vi "Get_Data_With_Condition.vi"(8 "error in (no error)":errorcluster caption="entrée d'erreur (pas d'erreur)", 11 "Firebase Benches en entrée":refnum<class "Firebase Benches P2193.lvclass">) -> (0 "error out":errorcluster caption="sortie d'erreur", 3 "Firebase Benches en sortie":refnum<class "Firebase Benches P2193.lvclass">)   [LabVIEW 2020, in "Library Instrument & Equipement.lvlib" / "Library FireBase.lvlib" / "Firebase Benches P2193.lvclass"]
doc: "Returns data according to Value_To_Find on Collection_to_find Use Nb_To_Read to determine the number to read\nPlease initialise the following values before use the VI\n - Name BDD\n - Value to find\n - API Key\n - Field Filter\n - Field Order\n - Collection_to_find\n\nIf there is no Field order -> Field Order=Field Filter"
uses:
  Firebase Benches P2193.lvclass
  C:/Users/ngarcin/OneDrive - Altyor/Standard TB/Class/Firebase/Source/Firebase Altyor/Firebase Altyor.lvclass
  C:/Users/ngarcin/OneDrive - Altyor/Standard TB/Class/Firebase/Source/Firebase Driver/Firebase Driver.lvclass
  Firebase Benches P2193.lvclass/Firebase Benches P2193.ctl
  JSON API/JSON Value/Set from JSON string.vi
  JSON API/JSON Value/JSON Value.lvclass
  Firebase Altyor/Firebase Altyor.lvclass
  JSON API/Variant JSON/Variant JSON.lvlib
  JSON API/Get Polymorphic/JSON GetSet.lvlib
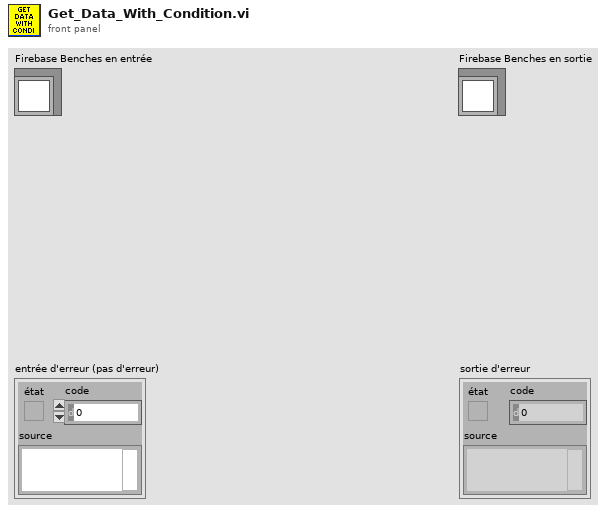
[diagram p1: front panel]
types:
  T1 = cluster{"name":string, "fields":cluster{"Result":cluster{"booleanValue":bool}, "CreationDate":cluster{"timestampValue":string}, "Batch":cluster{"stringValue":string}, "SerialNumber":cluster{"stringValue":string}, "EndOfProduction":cluster{"timestampValue":string}, "FW_Version":cluster{"mapValue":cluster{"fields":cluster{"Bootloader":cluster{"mapValue":cluster{"fields":cluster{"File_Name":cluster{"stringValue":string}, "Version":cluster{"mapValue":cluster{"fields":cluster{"Major":cluster{"stringValue":string}, "Minor":cluster{"stringValue":string}}}}, "Checksum":cluster{"stringValue":string}}}}, "SoftDevice":cluster{"mapValue":cluster{"fields":cluster{"File_Name":cluster{"stringValue":string}, "Version":cluster{"mapValue":cluster{"fields":cluster{"Major":cluster{"stringValue":string}, "Minor":cluster{"stringValue":string}}}}, "Checksum":cluster{"stringValue":string}}}}, "DFU":cluster{"mapValue":cluster{"fields":cluster{"File_Name":cluster{"stringValue":string}, "Version":cluster{"mapValue":cluster{"fields":cluster{"Major":cluster{"stringValue":string}, "Minor":cluster{"stringValue":string}}}}, "Checksum":cluster{"stringValue":string}}}}}}}, "PartNumber":cluster{"stringValue":string}, "OrderNumber":cluster{"stringValue":string}, "Operator":cluster{"stringValue":string}, "SN_CPU":cluster{"stringValue":string}}}[]
  T2 = cluster{"name":string, "fields":cluster{"Result":cluster{"booleanValue":bool}, "CreationDate":cluster{"timestampValue":string}, "Batch":cluster{"stringValue":string}, "SerialNumber":cluster{"stringValue":string}, "EndOfProduction":cluster{"timestampValue":string}, "FW_Version":cluster{"mapValue":cluster{"fields":cluster{"Bootloader":cluster{"mapValue":cluster{"fields":cluster{"File_Name":cluster{"stringValue":string}, "Version":cluster{"mapValue":cluster{"fields":cluster{"Major":cluster{"stringValue":string}, "Minor":cluster{"stringValue":string}}}}, "Checksum":cluster{"stringValue":string}}}}, "SoftDevice":cluster{"mapValue":cluster{"fields":cluster{"File_Name":cluster{"stringValue":string}, "Version":cluster{"mapValue":cluster{"fields":cluster{"Major":cluster{"stringValue":string}, "Minor":cluster{"stringValue":string}}}}, "Checksum":cluster{"stringValue":string}}}}, "DFU":cluster{"mapValue":cluster{"fields":cluster{"File_Name":cluster{"stringValue":string}, "Version":cluster{"mapValue":cluster{"fields":cluster{"Major":cluster{"stringValue":string}, "Minor":cluster{"stringValue":string}}}}, "Checksum":cluster{"stringValue":string}}}}}}}, "PartNumber":cluster{"stringValue":string}, "OrderNumber":cluster{"stringValue":string}, "Operator":cluster{"stringValue":string}, "SN_CPU":cluster{"stringValue":string}}}
  T3 = cluster{"document":cluster{"name":string, "fields":cluster{"Result":cluster{"booleanValue":bool}, "CreationDate":cluster{"timestampValue":string}, "Batch":cluster{"stringValue":string}, "SerialNumber":cluster{"stringValue":string}, "EndOfProduction":cluster{"timestampValue":string}, "FW_Version":cluster{"mapValue":cluster{"fields":cluster{"Bootloader":cluster{"mapValue":cluster{"fields":cluster{"File_Name":cluster{"stringValue":string}, "Version":cluster{"mapValue":cluster{"fields":cluster{"Major":cluster{"stringValue":string}, "Minor":cluster{"stringValue":string}}}}, "Checksum":cluster{"stringValue":string}}}}, "SoftDevice":cluster{"mapValue":cluster{"fields":cluster{"File_Name":cluster{"stringValue":string}, "Version":cluster{"mapValue":cluster{"fields":cluster{"Major":cluster{"stringValue":string}, "Minor":cluster{"stringValue":string}}}}, "Checksum":cluster{"stringValue":string}}}}, "DFU":cluster{"mapValue":cluster{"fields":cluster{"File_Name":cluster{"stringValue":string}, "Version":cluster{"mapValue":cluster{"fields":cluster{"Major":cluster{"stringValue":string}, "Minor":cluster{"stringValue":string}}}}, "Checksum":cluster{"stringValue":string}}}}}}}, "PartNumber":cluster{"stringValue":string}, "OrderNumber":cluster{"stringValue":string}, "Operator":cluster{"stringValue":string}, "SN_CPU":cluster{"stringValue":string}}}}
  T4 = cluster{"document":cluster{"name":string, "fields":cluster{"Result":cluster{"booleanValue":bool}, "CreationDate":cluster{"timestampValue":string}, "Batch":cluster{"stringValue":string}, "SerialNumber":cluster{"stringValue":string}, "EndOfProduction":cluster{"timestampValue":string}, "FW_Version":cluster{"mapValue":cluster{"fields":cluster{"Bootloader":cluster{"mapValue":cluster{"fields":cluster{"File_Name":cluster{"stringValue":string}, "Version":cluster{"mapValue":cluster{"fields":cluster{"Major":cluster{"stringValue":string}, "Minor":cluster{"stringValue":string}}}}, "Checksum":cluster{"stringValue":string}}}}, "SoftDevice":cluster{"mapValue":cluster{"fields":cluster{"File_Name":cluster{"stringValue":string}, "Version":cluster{"mapValue":cluster{"fields":cluster{"Major":cluster{"stringValue":string}, "Minor":cluster{"stringValue":string}}}}, "Checksum":cluster{"stringValue":string}}}}, "DFU":cluster{"mapValue":cluster{"fields":cluster{"File_Name":cluster{"stringValue":string}, "Version":cluster{"mapValue":cluster{"fields":cluster{"Major":cluster{"stringValue":string}, "Minor":cluster{"stringValue":string}}}}, "Checksum":cluster{"stringValue":string}}}}}}}, "PartNumber":cluster{"stringValue":string}, "OrderNumber":cluster{"stringValue":string}, "Operator":cluster{"stringValue":string}, "SN_CPU":cluster{"stringValue":string}}}}[]
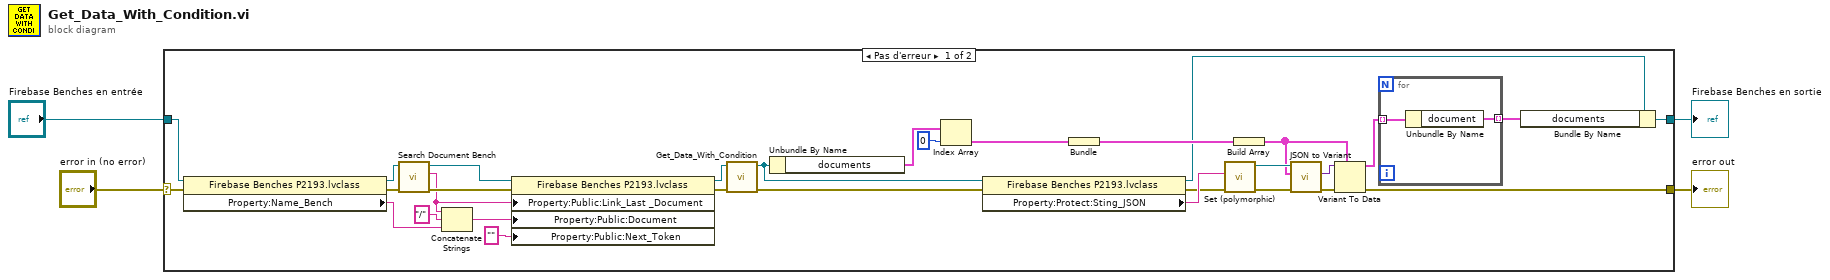
[diagram p0: block diagram]
diagram:
  n1 = case shown="Pas d'erreur" "error in (no error)" {
    selector: "error in (no error)" -> [w12 w39]
    tunnel: "Firebase Benches en entrée" -> [w10 w38]
    tunnel: [w5 w39] -> w3
    tunnel: [w13 w38] -> w2
    frame No Error {
      n2 = property class="Firebase Benches P2193.lvclass"(reference=w10, error in=w12) -> (reference out=w9:refnum<class "Firebase Benches P2193.lvclass">, error out=w11:errorcluster, "Property:Name_Bench"=w8:string)
      n3 = call "Search Document Bench.vi"("entrée d'erreur (pas d'erreur)"=w11, "Firebase Altyor en entrée"=w9) -> ("sortie d'erreur"=w35:errorcluster, "Source"=w33:string, "Firebase Altyor en sortie"=w34:refnum<class "Firebase Benches P2193.lvclass">)  [unwired: 7 in]
      n4 = Concatenate Strings(w33, "/" ("chaîne"), w8) -> (w32:string)
      n5 = property class="Firebase Benches P2193.lvclass"(reference=w34, error in=w35, "Property:Public:Link_Last _Document"=w33, "Property:Public:Document"=w32, "Property:Public:Next_Token"="" ("Next_Token")) -> (reference out=w28:refnum<class "Firebase Benches P2193.lvclass">, error out=w29:errorcluster)
      n6 = call-parent "Get_Data_With_Condition.vi"("error in (no error)"=w29, "Firebase Benches en entrée"=w28) -> ("error out"=w16:errorcluster, "Firebase Benches en sortie"=w15:refnum<class "Firebase Benches P2193.lvclass">)  [unwired: 8 in]
      n7 = Unbundle By Name(w15) -> ("documents"=w22:T1)
      n8 = Index Array(array=w22, index=0 ("indice")) -> (element=w20:T2)
      n9 = property class="Firebase Benches P2193.lvclass"(reference=w15, error in=w16) -> (reference out=w6:refnum<class "Firebase Benches P2193.lvclass">, error out=w14:errorcluster, "Property:Protect:Sting_JSON"=w23:string)
      n10 = Bundle("document"=w20) -> (w19:T3)  [unwired: 1 in]
      n11 = call-poly "Set (polymorphic).vi"("error in (no error)"=w14, "JSON stream"=w23) -> ("error out"=w24:errorcluster, "JSON Value out"=w26:refnum<class "JSON Value.lvclass">)  [unwired: 7 in, 1 out]
      n12 = Build Array(w19) -> (w18:T4)
      n13 = call "JSON to Variant.vi"("error in (no error)"=w24, "Variant (Data Type)"=w18, "JSON Value"=w26) -> ("error out"=w25:errorcluster, "Variant out"=w7:variant)  [unwired: 7 in]
      n14 = Variant To Data(error in=w25, type=w18, Variant=w7) -> (data=w17:T4, error out=w5:errorcluster)
      n15 = for {
        tunnel: w17 -> [w37] mode=indexing
        tunnel: [w36] -> w27 mode=indexing
        n16 = Unbundle By Name(w37) -> ("document"=w36:T2)
      }
      n17 = Bundle By Name(cluster=w6, "documents"=w27) -> (w13:refnum<class "Firebase Benches P2193.lvclass">)
    }
    frame Error {
    }
  }
  "error out" <- w3
  "Firebase Benches en sortie" <- w2
